vi "读取Pandoc路径.vi"(8 "error in (no error)":errorcluster caption="错误输入（无错误）", 11 "EPUB输入":refnum<class "EPUB.lvclass">) -> (0 "error out":errorcluster caption="错误输出", 2 "Pandoc路径":path, 3 "EPUB输出":refnum<class "EPUB.lvclass">)   [LabVIEW 2016]
uses:
  EPUB.lvclass
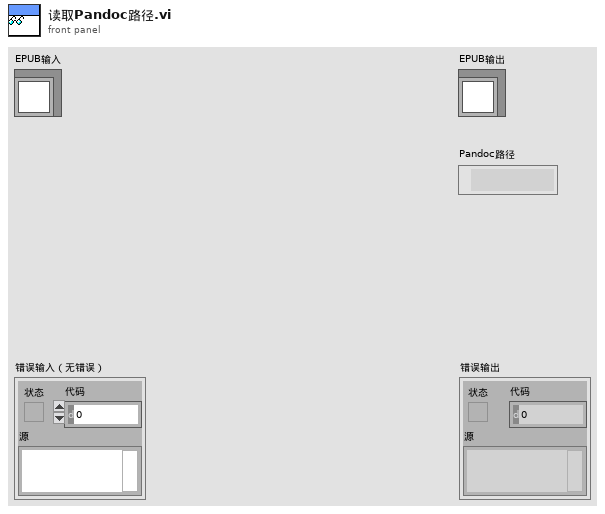
[diagram p1: front panel]
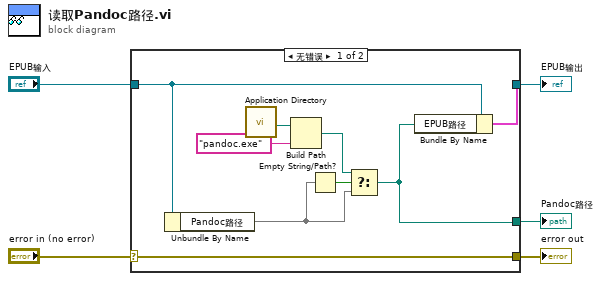
[diagram p0: block diagram]
diagram:
  n1 = case shown="无错误" "error in (no error)" {
    selector: "error in (no error)" -> [w14 w15]
    tunnel: [w14 w15] -> w4
    tunnel: [w7 w16] -> w2
    tunnel: "EPUB输入" -> [w13 w16]
    tunnel: [w6 _] -> w1
    frame No Error {
      n2 = Unbundle By Name(w13) -> ("Pandoc路径"=w11)
      n3 = call <vilib>:"Application Directory.vi"() -> ("Application Directory"=w10:path)
      n4 = Build Path(base path=w10, name or relative path="pandoc.exe" ("名称或相对路径")) -> (appended path=w8:path)
      n5 = Empty String/Path?(string/path=w11) -> (empty?=w12:bool)
      n6 = Select(t=w8, s=w12, f=w11) -> (s? t:f=w6:path)
      n7 = Bundle By Name(cluster=w13, "EPUB路径"=w6) -> (w7:cluster{})
    }
    frame Error {
    }
  }
  "error out" <- w4
  "EPUB输出" <- w2
  "Pandoc路径" <- w1
